vi "GetControlValue.vi"(0 "index":i32, 1 "Datatype":string, 5 "error in (no error)":errorcluster, 6 "Data":T1) -> (14 "Value":variant, 19 "error out":errorcluster)   [LabVIEW 2018]
uses:
  Ctrl/Data.ctl
  Ctrl/Caps.ctl
  Ctrl/Property.ctl
  Ctrl/PhysicalChannel.ctl
  Ctrl/Register.ctl
  Ctrl/Bitfield.ctl
  Ctrl/Scale.ctl
  Ctrl/ScaleType.ctl
  Ctrl/Enum.ctl
  Ctrl/EnumValue.ctl
  <vilib>/Utility/error.llb/DialogType.ctl
  API/Parser/Paser.lvlib
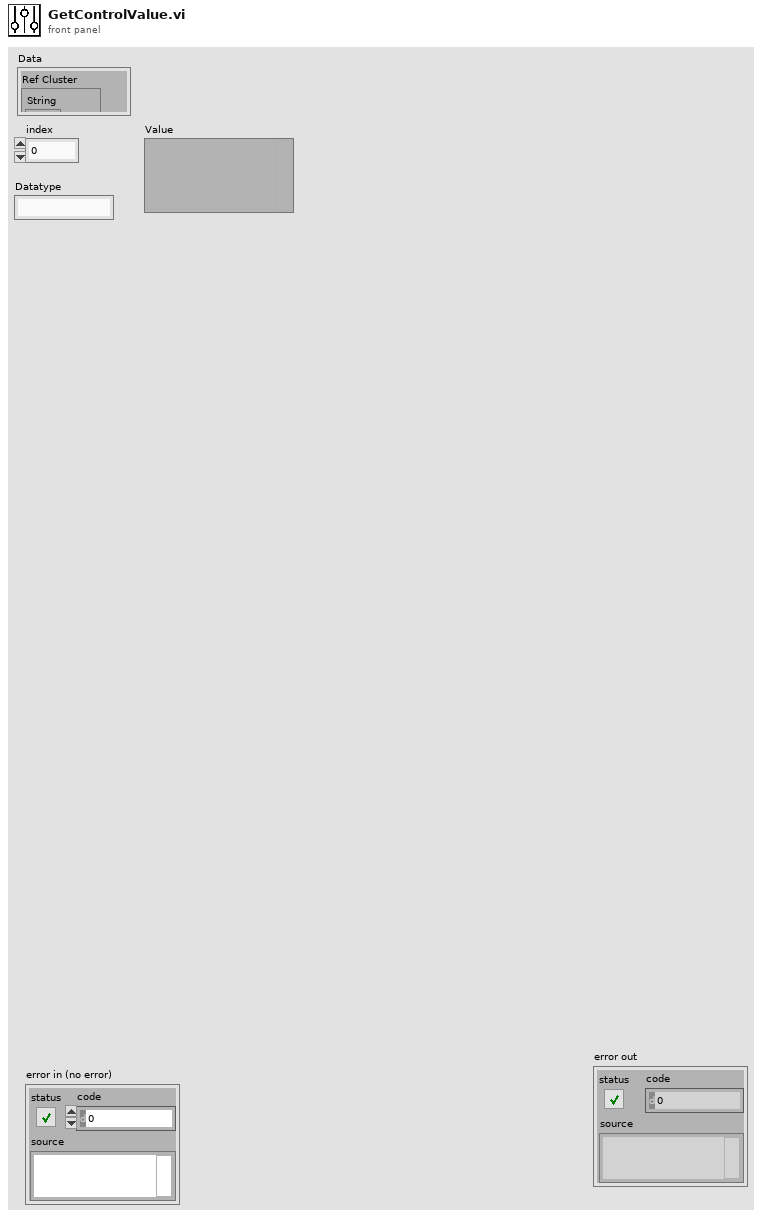
[diagram p1: front panel]
types:
  T1 = typedef "Data.ctl" = cluster{"Ref Cluster":cluster{"String":refnum<vi>, "U8":refnum<vi>, "I8":refnum<vi>, "U32":refnum<vi>, "I32":refnum<vi>, "U64":refnum<vi>, "I64":refnum<vi>, "Ring":refnum<vi>, "DBL":refnum<vi>, "Add":refnum<vi>, "Remove":refnum<vi>, "Property tree":refnum<vi>, "confirm":refnum<vi>}, "JSON Text":string, "Original JSON Text":string, "Caps":T2, "SLSC Output Tree":cluster{"Left Cell String":string, "Child Text":string[], "Child Tag":string, "Item Indent":i32, "Child Only?":bool, "Glyph Index":i32, "offline value":variant}[], "Ref Index and Control Type":cluster{"index":i32, "Datatype":string}, "Selected Type and name":cluster{"Selected Type":enum16{"Property", "Physical Channel", "Other"}, "Selected Property Name":string}, "Update whole Tree?":bool}
  T2 = typedef "Caps.ctl" = cluster{"properties":T3[], "physical channels":T4[], "registers":T5[], "scales":T7[], "enums":T9[], "productName":string}
  T3 = typedef "Property.ctl" = cluster{"name":string, "bitfield":string, "value":variant, "dataType":string, "min":variant, "max":variant, "scale":string, "access":string}
  T4 = typedef "PhysicalChannel.ctl" = cluster{"name":string, "properties":T3[]}
  T5 = typedef "Register.ctl" = cluster{"name":string, "address":i32, "size":i32, "bitfields":T6[], "initialValue":variant, "connectedProperties":string[]}
  T6 = typedef "Bitfield.ctl" = cluster{"name":string, "offset":i32, "size":i32, "signed":bool}
  T7 = typedef "Scale.ctl" = cluster{"name":string, "type":T8, "params":variant}
  T8 = typedef "ScaleType.ctl" = enum16{"NoScale", "Table", "Polynomial", "Linear"}
  T9 = typedef "Enum.ctl" = cluster{"name":string, "values":T10[]}
  T10 = typedef "EnumValue.ctl" = cluster{"name":string, "value":i32}
  T11 = cluster{"Left Cell String":string, "Child Text":string[], "Child Tag":string, "Item Indent":i32, "Child Only?":bool, "Glyph Index":i32, "offline value":variant}[]
  T12 = cluster{"String":refnum<vi>, "U8":refnum<vi>, "I8":refnum<vi>, "U32":refnum<vi>, "I32":refnum<vi>, "U64":refnum<vi>, "I64":refnum<vi>, "Ring":refnum<vi>, "DBL":refnum<vi>, "Add":refnum<vi>, "Remove":refnum<vi>, "Property tree":refnum<vi>, "confirm":refnum<vi>}
  T13 = typedef "DialogType.ctl" = u16
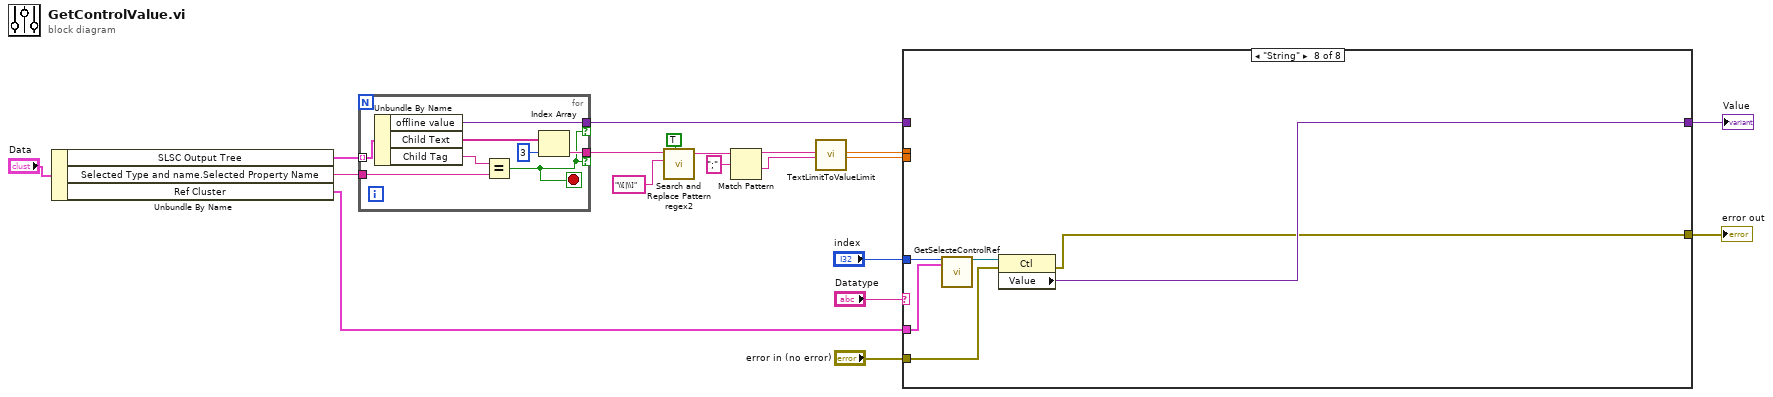
[diagram p0: block diagram]
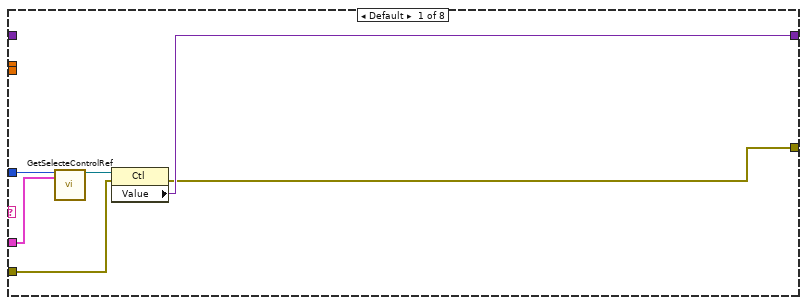
[diagram p2: hidden frame]
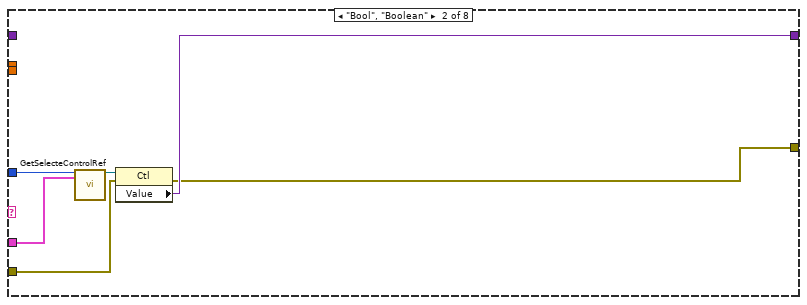
[diagram p3: hidden frame]
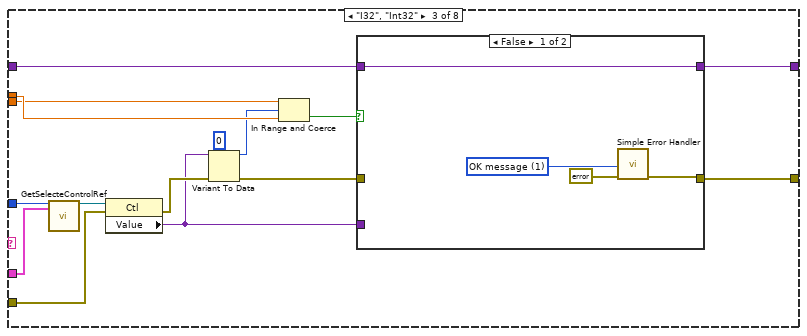
[diagram p4: hidden frame]
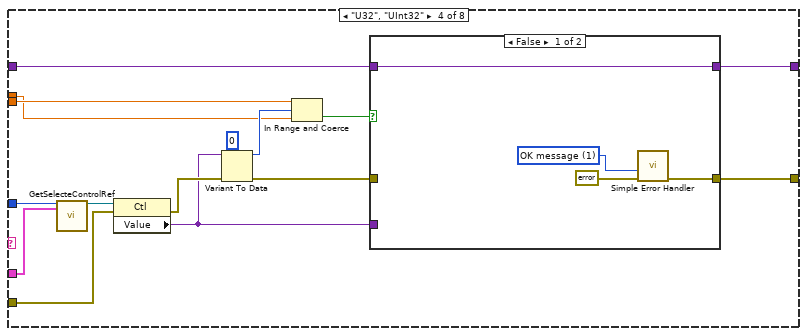
[diagram p6: hidden frame]
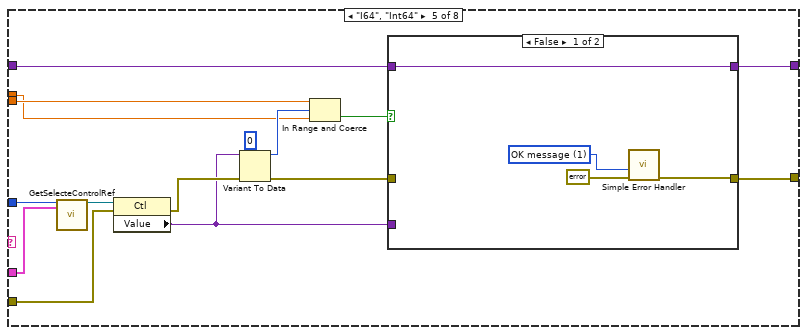
[diagram p8: hidden frame]
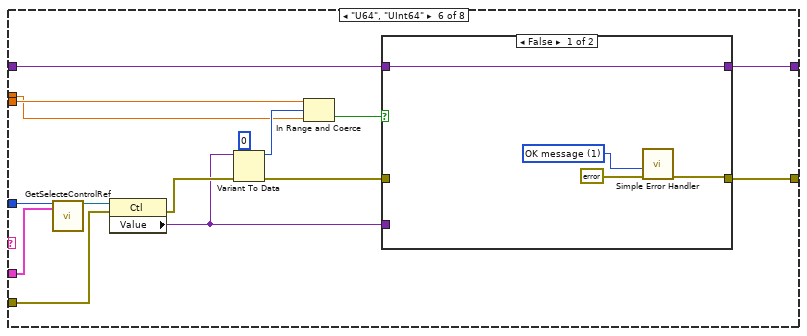
[diagram p10: hidden frame]
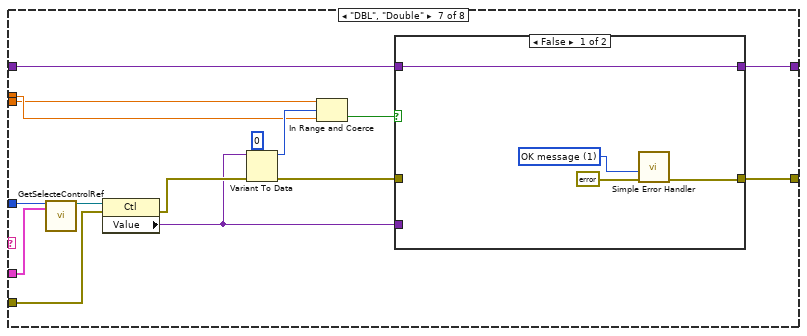
[diagram p12: hidden frame]
diagram:
  n1 = Unbundle By Name("Data") -> ("SLSC Output Tree"=w15:T11, "Selected Type and name.Selected Property Name"=w14:string, "Ref Cluster"=w1:T12)
  n2 = for {
    tunnel: w15 -> [w27] mode=indexing
    tunnel: w14 -> [w26]
    tunnel: [w23] -> w11 if=w20
    tunnel: [w21] -> w4 if=w20
    stop <- w20 stop-if-true
    n3 = Unbundle By Name(w27) -> ("offline value"=w21:variant, "Child Text"=w25:string[], "Child Tag"=w22:string)
    n4 = Equal?(x=w22, y=w26) -> (x = y?=w20:bool)
    n5 = Index Array(array=w25, index=3) -> (element=w23:string)
  }
  n6 = call "Search and Replace Pattern regex2.vi"("replace all? (F)"=TRUE, "regular expression (\"\")"="\\[|\\]" ("regular expression (\"\")"), "string"=w11) -> ("result string"=w10:string)  [unwired: 6 in, 2 out]
  n7 = Match Pattern(string=w10, regular expression=";") -> (before substring=w8:string, after substring=w7:string)  [unwired: 1 in, 2 out]
  n8 = call "TextLimitToValueLimit.vi"("min"=w8, "max"=w7) -> ("min"=w6:dbl, "max"=w5:dbl)  [unwired: 16 in]
  n9 = case shown="\"String\"" "Datatype" {
    tunnel: "index" -> [w33 w38 w53 w75 w96 w117 w138 w150]
    tunnel: w1 -> [w28 w37 w52 w74 w95 w116 w137 w149]
    tunnel: "error in (no error)" -> [w31 w36 w51 w72 w93 w114 w135 w147]
    tunnel: w6 -> [_ _ w50 w61 w82 w103 w125 _]
    tunnel: w5 -> [_ _ w49 w62 w83 w104 w124 _]
    tunnel: w4 -> [_ _ w44 w67 w88 w109 w130 _]
    tunnel: [w30 w35 w43 w66 w85 w106 w129 w146] -> w3
    tunnel: [w29 w34 w40 w65 w84 w105 w128 w145] -> w2
    frame Default {
      n10 = call "GetSelecteControlRef.vi"("index"=w33, "Ref Cluster"=w28) -> ("Control out"=w32:refnum<vi>)  [unwired: 17 in]
      n11 = property class="Ctl"(reference=w32, error in=w31) -> (error out=w29:errorcluster, "Value"=w30:variant)  [unwired: 1 out]
    }
    frame "Bool", "Boolean" {
      n12 = call "GetSelecteControlRef.vi"("index"=w38, "Ref Cluster"=w37) -> ("Control out"=w39:refnum<vi>)  [unwired: 17 in]
      n13 = property class="Ctl"(reference=w39, error in=w36) -> (error out=w34:errorcluster, "Value"=w35:variant)  [unwired: 1 out]
    }
    frame "I32", "Int32" {
      n14 = call "GetSelecteControlRef.vi"("index"=w53, "Ref Cluster"=w52) -> ("Control out"=w54:refnum<vi>)  [unwired: 17 in]
      n15 = property class="Ctl"(reference=w54, error in=w51) -> (error out=w46:errorcluster, "Value"=w42:variant)  [unwired: 1 out]
      n16 = Variant To Data(error in=w46, type=0, Variant=w42) -> (data=w47:i32, error out=w41:errorcluster)
      n17 = In Range and Coerce(upper limit=w49, x=w47, lower limit=w50) -> (In Range?=w45:bool)  [unwired: 1 out]
      n18 = case shown="False" w45 {
        tunnel: w44 -> [w58 _]
        tunnel: [w58 w60] -> w43
        tunnel: w42 -> [_ w60]
        tunnel: [w55 w59] -> w40
        tunnel: w41 -> [_ w59]
        frame False {
          w56 = T13 1 items=["no dialog", "OK message", "continue or stop message", "OK message + warnings", "continue/stop + warnings"] ("type of dialog (OK msg:1)")
          n19 = call <vilib>:"Simple Error Handler.vi"("type of dialog (OK msg:1)"=w56, "error in (no error)"=errorcluster {"status"=TRUE, "code"=-995, "source"="Input value out of min or max range"} ("error out")) -> ("error out"=w55:errorcluster)  [unwired: 3 in, 4 out]
        }
        frame True {
        }
      }
    }
    frame "U32", "UInt32" {
      n20 = call "GetSelecteControlRef.vi"("index"=w75, "Ref Cluster"=w74) -> ("Control out"=w73:refnum<vi>)  [unwired: 17 in]
      n21 = property class="Ctl"(reference=w73, error in=w72) -> (error out=w64:errorcluster, "Value"=w63:variant)  [unwired: 1 out]
      n22 = Variant To Data(error in=w64, type=0, Variant=w63) -> (data=w70:i32, error out=w68:errorcluster)
      n23 = In Range and Coerce(upper limit=w62, x=w70, lower limit=w61) -> (In Range?=w69:bool)  [unwired: 1 out]
      n24 = case shown="False" w69 {
        tunnel: w67 -> [w79 _]
        tunnel: [w79 w81] -> w66
        tunnel: w63 -> [_ w81]
        tunnel: [w76 w80] -> w65
        tunnel: w68 -> [_ w80]
        frame False {
          w77 = T13 1 items=["no dialog", "OK message", "continue or stop message", "OK message + warnings", "continue/stop + warnings"] ("type of dialog (OK msg:1)")
          n25 = call <vilib>:"Simple Error Handler.vi"("type of dialog (OK msg:1)"=w77, "error in (no error)"=errorcluster {"status"=TRUE, "code"=-995, "source"="Input value out of min or max range"} ("error out")) -> ("error out"=w76:errorcluster)  [unwired: 3 in, 4 out]
        }
        frame True {
        }
      }
    }
    frame "I64", "Int64" {
      n26 = call "GetSelecteControlRef.vi"("index"=w96, "Ref Cluster"=w95) -> ("Control out"=w94:refnum<vi>)  [unwired: 17 in]
      n27 = property class="Ctl"(reference=w94, error in=w93) -> (error out=w87:errorcluster, "Value"=w86:variant)  [unwired: 1 out]
      n28 = Variant To Data(error in=w87, type=0, Variant=w86) -> (data=w91:i32, error out=w89:errorcluster)
      n29 = In Range and Coerce(upper limit=w83, x=w91, lower limit=w82) -> (In Range?=w90:bool)  [unwired: 1 out]
      n30 = case shown="False" w90 {
        tunnel: w88 -> [w100 _]
        tunnel: [w100 w102] -> w85
        tunnel: w86 -> [_ w102]
        tunnel: [w97 w101] -> w84
        tunnel: w89 -> [_ w101]
        frame False {
          w98 = T13 1 items=["no dialog", "OK message", "continue or stop message", "OK message + warnings", "continue/stop + warnings"] ("type of dialog (OK msg:1)")
          n31 = call <vilib>:"Simple Error Handler.vi"("type of dialog (OK msg:1)"=w98, "error in (no error)"=errorcluster {"status"=TRUE, "code"=-995, "source"="Input value out of min or max range"} ("error out")) -> ("error out"=w97:errorcluster)  [unwired: 3 in, 4 out]
        }
        frame True {
        }
      }
    }
    frame "U64", "UInt64" {
      n32 = call "GetSelecteControlRef.vi"("index"=w117, "Ref Cluster"=w116) -> ("Control out"=w115:refnum<vi>)  [unwired: 17 in]
      n33 = property class="Ctl"(reference=w115, error in=w114) -> (error out=w108:errorcluster, "Value"=w107:variant)  [unwired: 1 out]
      n34 = Variant To Data(error in=w108, type=0, Variant=w107) -> (data=w112:i32, error out=w110:errorcluster)
      n35 = In Range and Coerce(upper limit=w104, x=w112, lower limit=w103) -> (In Range?=w111:bool)  [unwired: 1 out]
      n36 = case shown="False" w111 {
        tunnel: w109 -> [w121 _]
        tunnel: [w121 w123] -> w106
        tunnel: w107 -> [_ w123]
        tunnel: [w118 w122] -> w105
        tunnel: w110 -> [_ w122]
        frame False {
          w119 = T13 1 items=["no dialog", "OK message", "continue or stop message", "OK message + warnings", "continue/stop + warnings"] ("type of dialog (OK msg:1)")
          n37 = call <vilib>:"Simple Error Handler.vi"("type of dialog (OK msg:1)"=w119, "error in (no error)"=errorcluster {"status"=TRUE, "code"=-995, "source"="Input value out of min or max range"} ("error out")) -> ("error out"=w118:errorcluster)  [unwired: 3 in, 4 out]
        }
        frame True {
        }
      }
    }
    frame "DBL", "Double" {
      n38 = call "GetSelecteControlRef.vi"("index"=w138, "Ref Cluster"=w137) -> ("Control out"=w136:refnum<vi>)  [unwired: 17 in]
      n39 = property class="Ctl"(reference=w136, error in=w135) -> (error out=w127:errorcluster, "Value"=w126:variant)  [unwired: 1 out]
      n40 = Variant To Data(error in=w127, type=0, Variant=w126) -> (data=w133:i32, error out=w131:errorcluster)
      n41 = In Range and Coerce(upper limit=w124, x=w133, lower limit=w125) -> (In Range?=w132:bool)  [unwired: 1 out]
      n42 = case shown="False" w132 {
        tunnel: w130 -> [w142 _]
        tunnel: [w142 w144] -> w129
        tunnel: w126 -> [_ w144]
        tunnel: [w139 w143] -> w128
        tunnel: w131 -> [_ w143]
        frame False {
          w140 = T13 1 items=["no dialog", "OK message", "continue or stop message", "OK message + warnings", "continue/stop + warnings"] ("type of dialog (OK msg:1)")
          n43 = call <vilib>:"Simple Error Handler.vi"("type of dialog (OK msg:1)"=w140, "error in (no error)"=errorcluster {"status"=TRUE, "code"=-995, "source"="Input value out of min or max range"} ("error out")) -> ("error out"=w139:errorcluster)  [unwired: 3 in, 4 out]
        }
        frame True {
        }
      }
    }
    frame "String" {
      n44 = call "GetSelecteControlRef.vi"("index"=w150, "Ref Cluster"=w149) -> ("Control out"=w148:refnum<vi>)  [unwired: 17 in]
      n45 = property class="Ctl"(reference=w148, error in=w147) -> (error out=w145:errorcluster, "Value"=w146:variant)  [unwired: 1 out]
    }
  }
  "Value" <- w3
  "error out" <- w2
